vi "color_to_value.vi"(0 "Tab Control":enum32{"Page 1", "Page 2"}(tab)) -> ()   [LabVIEW 2019]
panel:
  in  "Click to chose Third Band Color":u32(ring)
  in  "Click to chose Fourth Band Color":i32(ring)=1
  in  "Click to chose Five Band Color":i64(ring)
  in  "Click to chose Six Band Color":u64(ring)
  in  "?":bool
  in  "6B":bool
  in  "5B":bool
  in  "4B":bool
  in  "3B":bool
  in  "Click to chose Second Band Color":u32(ring)
  in  "2B":bool
  in  "1B":bool
  in  "Click to chose Frist Band Color":u32(ring)
  out "?":dbl format="%#_6e"
  out "?":dbl format="%#_1f"
  out "?":dbl format="%#_1f"
  out "?":dbl format="%#_1f"
  out "L6":bool
  out "L5":bool
  out "L4":bool
  out "L3":bool
  out "L2":bool
  out "L1":bool
  out "?":string
  out "?":dbl format="%.0p"
  out "?":string
  out "N":dbl format="%.0p "
  out "?":dbl format="( %.0p "
  out "?":string
  in  "OK":bool
  # "Color                                                 Value"
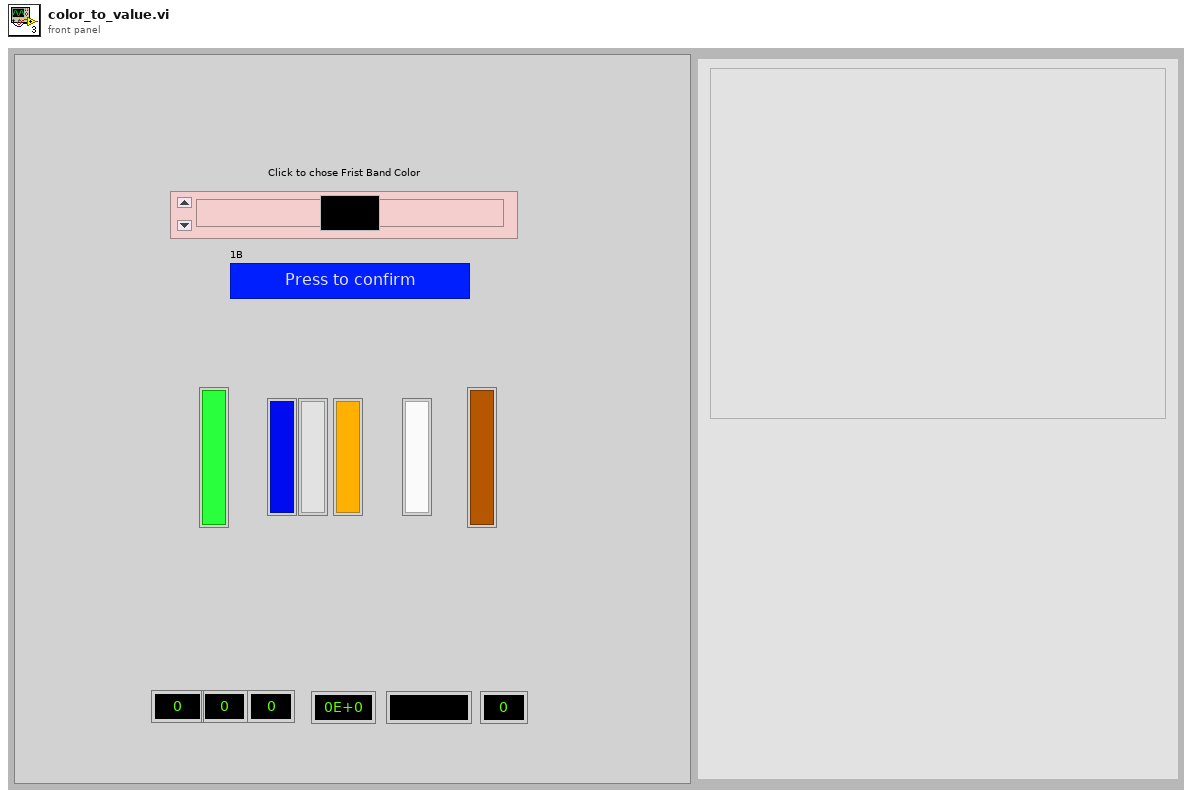
[diagram p1: front panel]
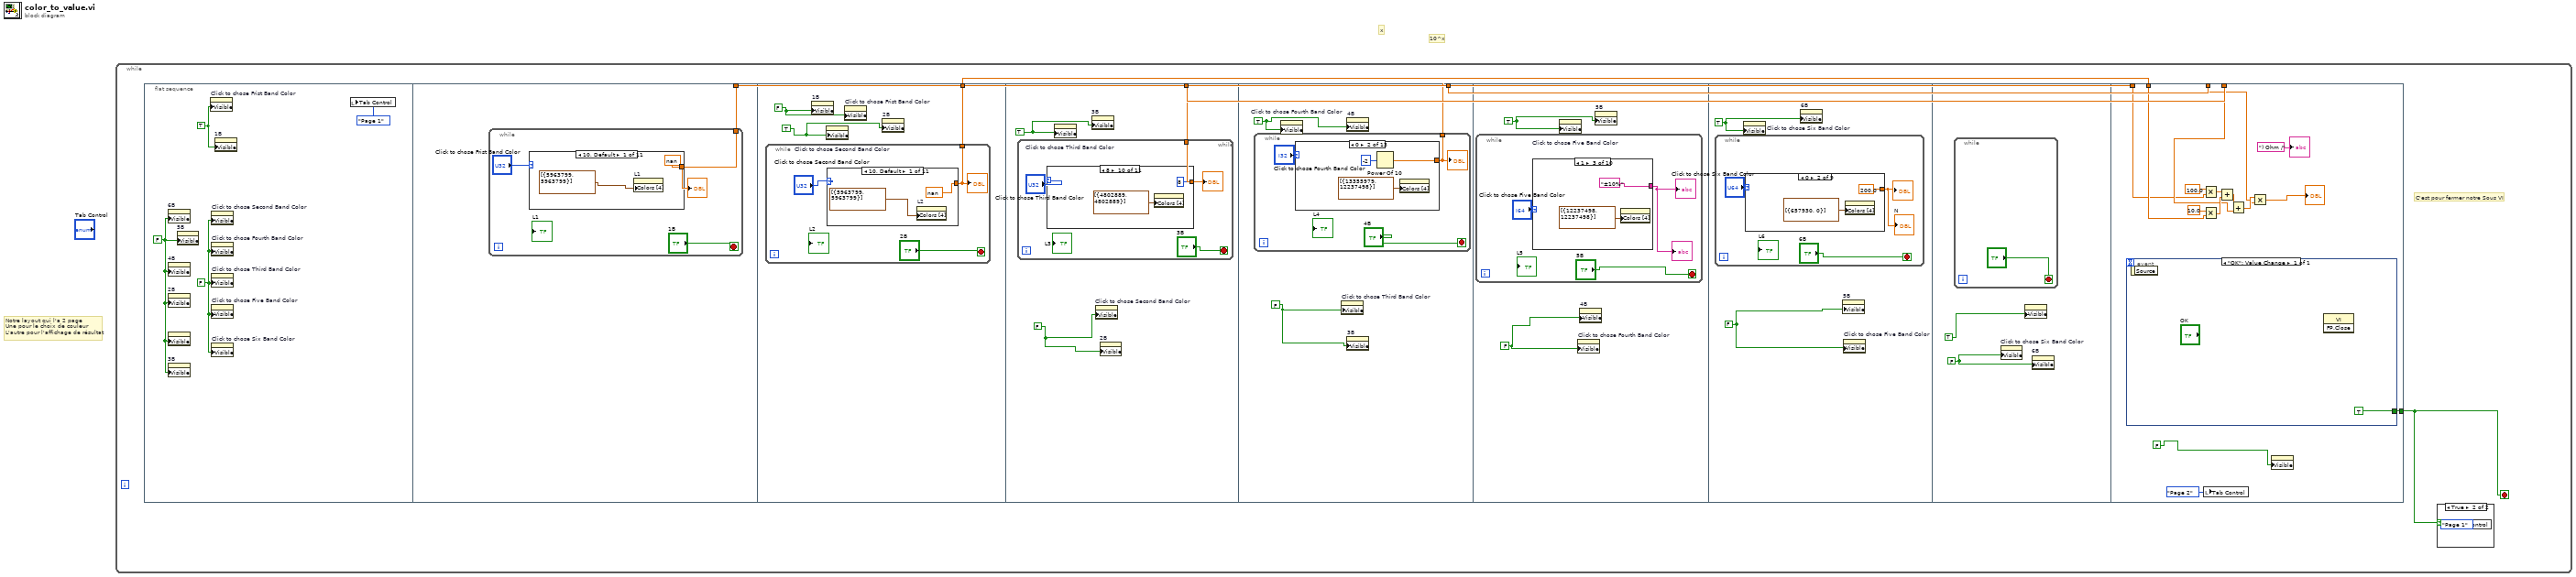
[diagram p0: block diagram]
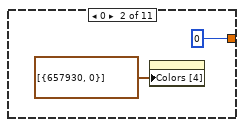
[diagram p3: hidden frame]
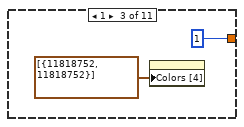
[diagram p4: hidden frame]
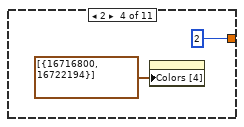
[diagram p5: hidden frame]
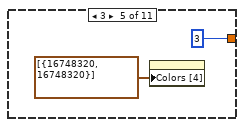
[diagram p6: hidden frame]
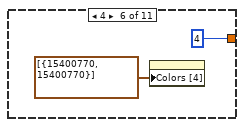
[diagram p7: hidden frame]
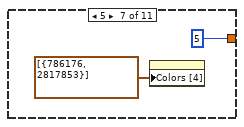
[diagram p8: hidden frame]
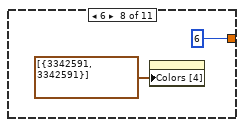
[diagram p9: hidden frame]
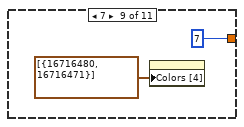
[diagram p10: hidden frame]
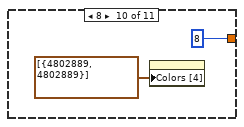
[diagram p11: hidden frame]
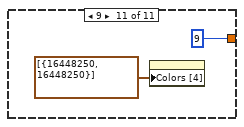
[diagram p12: hidden frame]
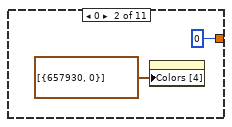
[diagram p13: hidden frame]
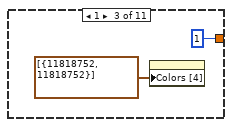
[diagram p14: hidden frame]
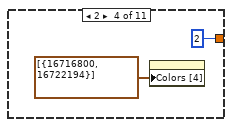
[diagram p15: hidden frame]
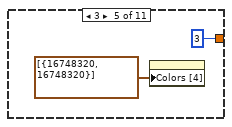
[diagram p16: hidden frame]
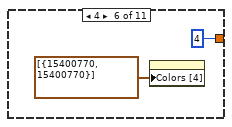
[diagram p17: hidden frame]
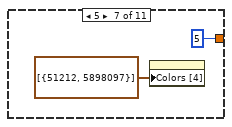
[diagram p18: hidden frame]
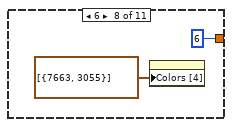
[diagram p19: hidden frame]
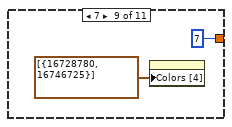
[diagram p20: hidden frame]
diagram:
  # "x"
  # "10^x"
  # "Notre layout qui l'a 2 page\nUne pour le choix de couleur\nL'autre pour l'affichage de résultat"
  n1 = while {
    stop <- w1 stop-if-true
    # "C'est pour fermer notre Sous VI"
    n2 = flat-sequence {
      tunnel: [w11] -> w4
      tunnel: [w39] -> w2
      tunnel: [w67] -> w5
      tunnel: [w95] -> w3
      tunnel: w4 -> [w191]
      tunnel: w3 -> [w195]
      tunnel: w5 -> [w194]
      tunnel: w2 -> [w193]
      tunnel: [w188] -> w1
      frame #0 {
        w9 = TRUE
        w8 = FALSE
        w10 = FALSE
        n3 = property on="6B" class="Bool"("Visible"=w8) -> ()  [unwired: 2 in, 2 out]
        n4 = property on="4B" class="Bool"("Visible"=w8) -> ()  [unwired: 2 in, 2 out]
        n5 = property on="2B" class="Bool"("Visible"=w8) -> ()  [unwired: 2 in, 2 out]
        n6 = property class="Bool"("Visible"=w8) -> ()  [unwired: 2 in, 2 out]
        n7 = property on="3B" class="Bool"("Visible"=w8) -> ()  [unwired: 2 in, 2 out]
        n8 = property on="5B" class="Bool"("Visible"=w8) -> ()  [unwired: 2 in, 2 out]
        n9 = property on="Click to chose Frist Band Color" class="Ring (strict)"("Visible"=w9) -> ()  [unwired: 2 in, 2 out]
        n10 = property on="Click to chose Second Band Color" class="Ring (strict)"("Visible"=w10) -> ()  [unwired: 2 in, 2 out]
        n11 = property on="Click to chose Fourth Band Color" class="Ring (strict)"("Visible"=w10) -> ()  [unwired: 2 in, 2 out]
        n12 = property on="Click to chose Third Band Color" class="Ring (strict)"("Visible"=w10) -> ()  [unwired: 2 in, 2 out]
        n13 = property on="Click to chose Five Band Color" class="Ring (strict)"("Visible"=w10) -> ()  [unwired: 2 in, 2 out]
        n14 = property on="Click to chose Six Band Color" class="Ring (strict)"("Visible"=w10) -> ()  [unwired: 2 in, 2 out]
        n15 = property on="1B" class="Bool"("Visible"=w9) -> ()  [unwired: 2 in, 2 out]
        n16 = local write "Tab Control"(enum32{"Page 1", "Page 2"}."Page 1" ("Tab Control")) -> ()
      }
      frame #1 {
        n17 = while {
          tunnel: [w13] -> w11
          stop <- "1B" stop-if-true
          n18 = case shown="10, Default" "Click to chose Frist Band Color" {
            tunnel: [nan 0 1 2 3 4 5 6 7 8 9] -> w13
            frame 10, Default {
              n19 = property on="L1" class="Bool (strict)"("Colors [4]"=cluster{u32, u32}[] [{5963799, 5963799}]) -> ()  [unwired: 2 in, 2 out]
            }
            frame 0 {
              n20 = property on="L1" class="Bool (strict)"("Colors [4]"=cluster{u32, u32}[] [{657930, 0}]) -> ()  [unwired: 2 in, 2 out]
            }
            frame 1 {
              n21 = property on="L1" class="Bool (strict)"("Colors [4]"=cluster{u32, u32}[] [{11818752, 11818752}]) -> ()  [unwired: 2 in, 2 out]
            }
            frame 2 {
              n22 = property on="L1" class="Bool (strict)"("Colors [4]"=cluster{u32, u32}[] [{16716800, 16722194}]) -> ()  [unwired: 2 in, 2 out]
            }
            frame 3 {
              n23 = property on="L1" class="Bool (strict)"("Colors [4]"=cluster{u32, u32}[] [{16748320, 16748320}]) -> ()  [unwired: 2 in, 2 out]
            }
            frame 4 {
              n24 = property on="L1" class="Bool (strict)"("Colors [4]"=cluster{u32, u32}[] [{15400770, 15400770}]) -> ()  [unwired: 2 in, 2 out]
            }
            frame 5 {
              n25 = property on="L1" class="Bool (strict)"("Colors [4]"=cluster{u32, u32}[] [{786176, 2817853}]) -> ()  [unwired: 2 in, 2 out]
            }
            frame 6 {
              n26 = property on="L1" class="Bool (strict)"("Colors [4]"=cluster{u32, u32}[] [{3342591, 3342591}]) -> ()  [unwired: 2 in, 2 out]
            }
            frame 7 {
              n27 = property on="L1" class="Bool (strict)"("Colors [4]"=cluster{u32, u32}[] [{16716480, 16716471}]) -> ()  [unwired: 2 in, 2 out]
            }
            frame 8 {
              n28 = property on="L1" class="Bool (strict)"("Colors [4]"=cluster{u32, u32}[] [{4802889, 4802889}]) -> ()  [unwired: 2 in, 2 out]
            }
            frame 9 {
              n29 = property on="L1" class="Bool (strict)"("Colors [4]"=cluster{u32, u32}[] [{16448250, 16448250}]) -> ()  [unwired: 2 in, 2 out]
            }
          }
          "?" <- w13
        }
      }
      frame #2 {
        w37 = FALSE
        w38 = TRUE
        n30 = while {
          tunnel: [w41] -> w39
          stop <- "2B" stop-if-true
          n31 = case shown="10, Default" "Click to chose Second Band Color" {
            tunnel: [nan 0 1 2 3 4 5 6 7 8 9] -> w41
            frame 10, Default {
              n32 = property on="L2" class="Bool (strict)"("Colors [4]"=cluster{u32, u32}[] [{5963799, 5963799}]) -> ()  [unwired: 2 in, 2 out]
            }
            frame 0 {
              n33 = property on="L2" class="Bool (strict)"("Colors [4]"=cluster{u32, u32}[] [{657930, 0}]) -> ()  [unwired: 2 in, 2 out]
            }
            frame 1 {
              n34 = property on="L2" class="Bool (strict)"("Colors [4]"=cluster{u32, u32}[] [{11818752, 11818752}]) -> ()  [unwired: 2 in, 2 out]
            }
            frame 2 {
              n35 = property on="L2" class="Bool (strict)"("Colors [4]"=cluster{u32, u32}[] [{16716800, 16722194}]) -> ()  [unwired: 2 in, 2 out]
            }
            frame 3 {
              n36 = property on="L2" class="Bool (strict)"("Colors [4]"=cluster{u32, u32}[] [{16748320, 16748320}]) -> ()  [unwired: 2 in, 2 out]
            }
            frame 4 {
              n37 = property on="L2" class="Bool (strict)"("Colors [4]"=cluster{u32, u32}[] [{15400770, 15400770}]) -> ()  [unwired: 2 in, 2 out]
            }
            frame 5 {
              n38 = property on="L2" class="Bool (strict)"("Colors [4]"=cluster{u32, u32}[] [{51212, 5898097}]) -> ()  [unwired: 2 in, 2 out]
            }
            frame 6 {
              n39 = property on="L2" class="Bool (strict)"("Colors [4]"=cluster{u32, u32}[] [{7663, 3055}]) -> ()  [unwired: 2 in, 2 out]
            }
            frame 7 {
              n40 = property on="L2" class="Bool (strict)"("Colors [4]"=cluster{u32, u32}[] [{16728780, 16746725}]) -> ()  [unwired: 2 in, 2 out]
            }
            frame 8 {
              n41 = property on="L2" class="Bool (strict)"("Colors [4]"=cluster{u32, u32}[] [{4802889, 4802889}]) -> ()  [unwired: 2 in, 2 out]
            }
            frame 9 {
              n42 = property on="L2" class="Bool (strict)"("Colors [4]"=cluster{u32, u32}[] [{16777215, 16777215}]) -> ()  [unwired: 2 in, 2 out]
            }
          }
          "?" <- w41
        }
        n43 = property on="1B" class="Bool"("Visible"=w37) -> ()  [unwired: 2 in, 2 out]
        n44 = property on="Click to chose Second Band Color" class="Ring (strict)"("Visible"=w38) -> ()  [unwired: 2 in, 2 out]
        n45 = property on="Click to chose Frist Band Color" class="Ring (strict)"("Visible"=w37) -> ()  [unwired: 2 in, 2 out]
        n46 = property on="2B" class="Bool"("Visible"=w38) -> ()  [unwired: 2 in, 2 out]
      }
      frame #3 {
        w65 = FALSE
        w66 = TRUE
        n47 = while {
          tunnel: [w69] -> w67
          stop <- "3B" stop-if-true
          n48 = case shown="8" "Click to chose Third Band Color" {
            tunnel: [nan 0 1 2 3 4 5 6 7 8 9] -> w69
            frame 10, Default {
              n49 = property on="L3" class="Bool (strict)"("Colors [4]"=cluster{u32, u32}[] [{5963799, 5963799}]) -> ()  [unwired: 2 in, 2 out]
            }
            frame 0 {
              n50 = property on="L3" class="Bool (strict)"("Colors [4]"=cluster{u32, u32}[] [{1513239, 197379}]) -> ()  [unwired: 2 in, 2 out]
            }
            frame 1 {
              n51 = property on="L3" class="Bool (strict)"("Colors [4]"=cluster{u32, u32}[] [{13136128, 13136128}]) -> ()  [unwired: 2 in, 2 out]
            }
            frame 2 {
              n52 = property on="L3" class="Bool (strict)"("Colors [4]"=cluster{u32, u32}[] [{16711699, 16728656}]) -> ()  [unwired: 2 in, 2 out]
            }
            frame 3 {
              n53 = property on="L3" class="Bool (strict)"("Colors [4]"=cluster{u32, u32}[] [{16684321, 16684321}]) -> ()  [unwired: 2 in, 2 out]
            }
            frame 4 {
              n54 = property on="L3" class="Bool (strict)"("Colors [4]"=cluster{u32, u32}[] [{16056130, 15400704}]) -> ()  [unwired: 2 in, 2 out]
            }
            frame 5 {
              n55 = property on="L3" class="Bool (strict)"("Colors [4]"=cluster{u32, u32}[] [{2027264, 6618880}]) -> ()  [unwired: 2 in, 2 out]
            }
            frame 6 {
              n56 = property on="L3" class="Bool (strict)"("Colors [4]"=cluster{u32, u32}[] [{16860, 16860}]) -> ()  [unwired: 2 in, 2 out]
            }
            frame 7 {
              n57 = property on="L3" class="Bool (strict)"("Colors [4]"=cluster{u32, u32}[] [{16734701, 14418097}]) -> ()  [unwired: 2 in, 2 out]
            }
            frame 8 {
              n58 = property on="L3" class="Bool (strict)"("Colors [4]"=cluster{u32, u32}[] [{4802889, 4802889}]) -> ()  [unwired: 2 in, 2 out]
            }
            frame 9 {
              n59 = property on="L3" class="Bool (strict)"("Colors [4]"=cluster{u32, u32}[] [{16777225, 16777225}]) -> ()  [unwired: 2 in, 2 out]
            }
          }
          "?" <- w69
        }
        n60 = property on="Click to chose Third Band Color" class="Ring (strict)"("Visible"=w66) -> ()  [unwired: 2 in, 2 out]
        n61 = property on="3B" class="Bool"("Visible"=w66) -> ()  [unwired: 2 in, 2 out]
        n62 = property on="Click to chose Second Band Color" class="Ring (strict)"("Visible"=w65) -> ()  [unwired: 2 in, 2 out]
        n63 = property on="2B" class="Bool"("Visible"=w65) -> ()  [unwired: 2 in, 2 out]
      }
      frame #4 {
        w93 = FALSE
        w94 = TRUE
        n64 = while {
          tunnel: [w97] -> w95
          stop <- "4B" stop-if-true
          n65 = case shown="0" "Click to chose Fourth Band Color" {
            tunnel: [1.0 w101 w104 w107 w110 w113 w116 w119 w122 w125 w128 w131 w134] -> w97
            frame 12, Default {
              n66 = property on="L4" class="Bool (strict)"("Colors [4]"=cluster{u32, u32}[] [{5963799, 5963799}]) -> ()  [unwired: 2 in, 2 out]
            }
            frame 0 {
              n67 = Power Of 10(x=-2) -> (10^x=w101:dbl)
              n68 = property on="L4" class="Bool (strict)"("Colors [4]"=cluster{u32, u32}[] [{13355979, 12237498}]) -> ()  [unwired: 2 in, 2 out]
            }
            frame 1 {
              n69 = Power Of 10(x=-1) -> (10^x=w104:dbl)
              n70 = property on="L4" class="Bool (strict)"("Colors [4]"=cluster{u32, u32}[] [{16763714, 16756736}]) -> ()  [unwired: 2 in, 2 out]
            }
            frame 2 {
              n71 = property on="L4" class="Bool (strict)"("Colors [4]"=cluster{u32, u32}[] [{0, 263172}]) -> ()  [unwired: 2 in, 2 out]
              n72 = Power Of 10(x=0) -> (10^x=w107:dbl)
            }
            frame 3 {
              n73 = property on="L4" class="Bool (strict)"("Colors [4]"=cluster{u32, u32}[] [{13128704, 13128704}]) -> ()  [unwired: 2 in, 2 out]
              n74 = Power Of 10(x=1) -> (10^x=w110:dbl)
            }
            frame 4 {
              n75 = property on="L4" class="Bool (strict)"("Colors [4]"=cluster{u32, u32}[] [{16716800, 16722194}]) -> ()  [unwired: 2 in, 2 out]
              n76 = Power Of 10(x=2) -> (10^x=w113:dbl)
            }
            frame 5 {
              n77 = property on="L4" class="Bool (strict)"("Colors [4]"=cluster{u32, u32}[] [{16748320, 16748320}]) -> ()  [unwired: 2 in, 2 out]
              n78 = Power Of 10(x=3) -> (10^x=w116:dbl)
            }
            frame 6 {
              n79 = property on="L4" class="Bool (strict)"("Colors [4]"=cluster{u32, u32}[] [{15400770, 15400770}]) -> ()  [unwired: 2 in, 2 out]
              n80 = Power Of 10(x=4) -> (10^x=w119:dbl)
            }
            frame 7 {
              n81 = property on="L4" class="Bool (strict)"("Colors [4]"=cluster{u32, u32}[] [{786176, 2817853}]) -> ()  [unwired: 2 in, 2 out]
              n82 = Power Of 10(x=5) -> (10^x=w122:dbl)
            }
            frame 8 {
              n83 = property on="L4" class="Bool (strict)"("Colors [4]"=cluster{u32, u32}[] [{3342591, 3342591}]) -> ()  [unwired: 2 in, 2 out]
              n84 = Power Of 10(x=6) -> (10^x=w125:dbl)
            }
            frame 9 {
              n85 = property on="L4" class="Bool (strict)"("Colors [4]"=cluster{u32, u32}[] [{16716480, 16716471}]) -> ()  [unwired: 2 in, 2 out]
              n86 = Power Of 10(x=7) -> (10^x=w128:dbl)
            }
            frame 10 {
              n87 = property on="L4" class="Bool (strict)"("Colors [4]"=cluster{u32, u32}[] [{4802889, 4802889}]) -> ()  [unwired: 2 in, 2 out]
              n88 = Power Of 10(x=8) -> (10^x=w131:dbl)
            }
            frame 11 {
              n89 = property on="L4" class="Bool (strict)"("Colors [4]"=cluster{u32, u32}[] [{16448250, 16448250}]) -> ()  [unwired: 2 in, 2 out]
              n90 = Power Of 10(x=9) -> (10^x=w134:dbl)
            }
          }
          "?" <- w97
        }
        n91 = property on="Click to chose Fourth Band Color" class="Ring (strict)"("Visible"=w94) -> ()  [unwired: 2 in, 2 out]
        n92 = property on="Click to chose Third Band Color" class="Ring (strict)"("Visible"=w93) -> ()  [unwired: 2 in, 2 out]
        n93 = property on="4B" class="Bool"("Visible"=w94) -> ()  [unwired: 2 in, 2 out]
        n94 = property on="3B" class="Bool"("Visible"=w93) -> ()  [unwired: 2 in, 2 out]
      }
      frame #5 {
        w138 = FALSE
        w137 = TRUE
        n95 = while {
          stop <- "5B" stop-if-true
          n96 = case shown="1" "Click to chose Five Band Color" {
            tunnel: ["±00%" "±20%" "±10%" "±5%" "±1%" "±2%" "±0,5%" "±0,25%" "±0,10%" "±0,05%"] -> w139
            frame 9, Default {
              n97 = property on="L5" class="Bool (strict)"("Colors [4]"=cluster{u32, u32}[] [{5963799, 5963799}]) -> ()  [unwired: 2 in, 2 out]
            }
            frame 0 {
              n98 = property on="L5" class="Bool (strict)"("Colors [4]"=cluster{u32, u32}[] [{16448250, 16448250}]) -> ()  [unwired: 2 in, 2 out]
            }
            frame 1 {
              n99 = property on="L5" class="Bool (strict)"("Colors [4]"=cluster{u32, u32}[] [{12237498, 12237498}]) -> ()  [unwired: 2 in, 2 out]
            }
            frame 2 {
              (unwired) 2.0
              n100 = property on="L5" class="Bool (strict)"("Colors [4]"=cluster{u32, u32}[] [{16366338, 16366338}]) -> ()  [unwired: 2 in, 2 out]
            }
            frame 3 {
              n101 = property on="L5" class="Bool (strict)"("Colors [4]"=cluster{u32, u32}[] [{13128704, 13128704}]) -> ()  [unwired: 2 in, 2 out]
            }
            frame 4 {
              n102 = property on="L5" class="Bool (strict)"("Colors [4]"=cluster{u32, u32}[] [{16716800, 16722194}]) -> ()  [unwired: 2 in, 2 out]
            }
            frame 5 {
              n103 = property on="L5" class="Bool (strict)"("Colors [4]"=cluster{u32, u32}[] [{3079978, 3079978}]) -> ()  [unwired: 2 in, 2 out]
            }
            frame 6 {
              n104 = property on="L5" class="Bool (strict)"("Colors [4]"=cluster{u32, u32}[] [{458911, 327880}]) -> ()  [unwired: 2 in, 2 out]
            }
            frame 7 {
              n105 = property on="L5" class="Bool (strict)"("Colors [4]"=cluster{u32, u32}[] [{16711894, 15663313}]) -> ()  [unwired: 2 in, 2 out]
            }
            frame 8 {
              n106 = property on="L5" class="Bool (strict)"("Colors [4]"=cluster{u32, u32}[] [{4802889, 4802889}]) -> ()  [unwired: 2 in, 2 out]
            }
          }
          "?" <- w139
          "?" <- w139
        }
        n107 = property on="Click to chose Five Band Color" class="Ring (strict)"("Visible"=w137) -> ()  [unwired: 2 in, 2 out]
        n108 = property on="Click to chose Fourth Band Color" class="Ring (strict)"("Visible"=w138) -> ()  [unwired: 2 in, 2 out]
        n109 = property on="4B" class="Bool"("Visible"=w138) -> ()  [unwired: 2 in, 2 out]
        n110 = property on="5B" class="Bool"("Visible"=w137) -> ()  [unwired: 2 in, 2 out]
      }
      frame #6 {
        w162 = FALSE
        w163 = TRUE
        n111 = while {
          stop <- "6B" stop-if-true
          n112 = case shown="0" "Click to chose Six Band Color" {
            tunnel: [0.0 200.0 100.0 50.0 15.0 25.0 10.0 5.0 1.0] -> w164
            frame 8, Default {
              n113 = property on="L6" class="Bool (strict)"("Colors [4]"=cluster{u32, u32}[] [{5963799, 5963799}]) -> ()  [unwired: 2 in, 2 out]
            }
            frame 0 {
              n114 = property on="L6" class="Bool (strict)"("Colors [4]"=cluster{u32, u32}[] [{657930, 0}]) -> ()  [unwired: 2 in, 2 out]
            }
            frame 1 {
              n115 = property on="L6" class="Bool (strict)"("Colors [4]"=cluster{u32, u32}[] [{11818752, 11818752}]) -> ()  [unwired: 2 in, 2 out]
            }
            frame 2 {
              n116 = property on="L6" class="Bool (strict)"("Colors [4]"=cluster{u32, u32}[] [{16716800, 16722194}]) -> ()  [unwired: 2 in, 2 out]
            }
            frame 3 {
              n117 = property on="L6" class="Bool (strict)"("Colors [4]"=cluster{u32, u32}[] [{16748320, 16748320}]) -> ()  [unwired: 2 in, 2 out]
            }
            frame 4 {
              n118 = property on="L6" class="Bool (strict)"("Colors [4]"=cluster{u32, u32}[] [{15400770, 15400770}]) -> ()  [unwired: 2 in, 2 out]
            }
            frame 5 {
              n119 = property on="L6" class="Bool (strict)"("Colors [4]"=cluster{u32, u32}[] [{393471, 6380031}]) -> ()  [unwired: 2 in, 2 out]
            }
            frame 6 {
              n120 = property on="L6" class="Bool (strict)"("Colors [4]"=cluster{u32, u32}[] [{16716480, 16711885}]) -> ()  [unwired: 2 in, 2 out]
            }
            frame 7 {
              n121 = property on="L6" class="Bool (strict)"("Colors [4]"=cluster{u32, u32}[] [{4802889, 4802889}]) -> ()  [unwired: 2 in, 2 out]
            }
          }
          "?" <- w164
          "N" <- w164
        }
        n122 = property on="Click to chose Six Band Color" class="Ring (strict)"("Visible"=w163) -> ()  [unwired: 2 in, 2 out]
        n123 = property on="6B" class="Bool"("Visible"=w163) -> ()  [unwired: 2 in, 2 out]
        n124 = property on="5B" class="Bool"("Visible"=w162) -> ()  [unwired: 2 in, 2 out]
        n125 = property on="Click to chose Five Band Color" class="Ring (strict)"("Visible"=w162) -> ()  [unwired: 2 in, 2 out]
      }
      frame #7 {
        w185 = FALSE
        n126 = while {
          stop <- "?" stop-if-true
        }
        n127 = property on="Click to chose Six Band Color" class="Ring (strict)"("Visible"=w185) -> ()  [unwired: 2 in, 2 out]
        n128 = property class="Bool"("Visible"=TRUE) -> ()  [unwired: 2 in, 2 out]
        n129 = property on="6B" class="Bool"("Visible"=w185) -> ()  [unwired: 2 in, 2 out]
      }
      frame #8 {
        n130 = event shown="[0] \"OK\": Value Change" {
          selector: _ -> [_]
          dyn-events: _ -> [_]
          timeout: _ -> [_]
          tunnel: [TRUE] -> w188
          event "OK": Value Change {
            n131 = event-data() -> ()  [unwired: 1 in, 1 out]
            n132 = invoke class="VI" method="FP.Close"() -> ()  [unwired: 3 in, 3 out]
          }
        }
        n133 = Multiply(x=100.0, y=w191) -> (x*y=w199:dbl)
        n134 = Multiply(x=10.0, y=w193) -> (x*y=w198:dbl)
        n135 = local write "Tab Control"(enum32{"Page 1", "Page 2"}."Page 2" ("Tab Control")) -> ()
        n136 = Add(x=w199, y=w198) -> (x+y=w197:dbl)
        n137 = Add(x=w197, y=w194) -> (x+y=w196:dbl)
        n138 = Multiply(x=w196, y=w195) -> (x*y=→"?":dbl)
        n139 = property class="Bool"("Visible"=FALSE) -> ()  [unwired: 2 in, 2 out]
        "?" <- ") Ohm /"
      }
    }
    n140 = case shown="True" w1 {
      frame False {
      }
      frame True {
        n141 = local write "Tab Control"(enum32{"Page 1", "Page 2"}."Page 1" ("Tab Control")) -> ()
      }
    }
  }
